vi "RES.vi"(0 "System no.":i32=1 min=1 max=4 step=1, 2 "Axes to reset":string[](array[string]), 5 "error in":errorcluster) -> (19 "error out":errorcluster)   [LabVIEW 2026]
doc: "RES (Reset Axis)\n\nDescription\nClears the \"Error\" bit (bit 0) in the status register of the axis (p. 97) and passes the axis from the \nFault state to the Ready to switch on state.\nFor further details, see \"Drive State Machine\" (p. 101). \n\nFormat\nRES <AxisID>\n\nArguments\n<AxisID>\nAn axis of the controller\nThe response to USG? CMD RES indicates in the #Related Units block for which axes the \ncommand can be used.\nPossible values: Alias of the axis (p. 94) \n\nResponse\nnone\n\nNotes\nThe status register of the axis can be queried with the STV? command (p. 66). \n\nUser command level\nUSR"
panel:
  # "RES (Reset Axis)\n\nClears the \"Error\" bit (bit 0) in the status register of the axis and passes the axis from the  Fault state to the Ready to switch on state.\nFor further details, see \"Drive State Machine\"."
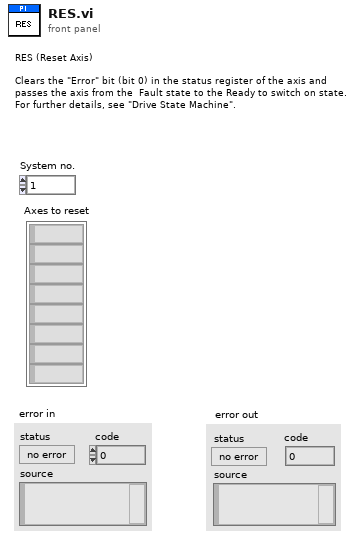
[diagram p1: front panel]
types:
  T1 = typedef "Syntax.ctl" = enum16{"GCS 1.0", "GCS 2.0", "GCS 3.0"}
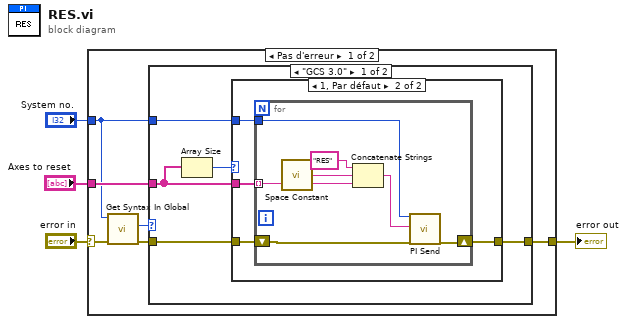
[diagram p0: block diagram]
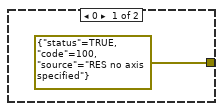
[diagram p2: hidden frame]
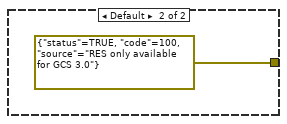
[diagram p3: hidden frame]
diagram:
  n1 = case shown="Pas d'erreur" "error in" {
    selector: "error in" -> [w8 w29]
    tunnel: [w10 w29] -> w4
    tunnel: "System no." -> [w5 _]
    tunnel: "Axes to reset" -> [w9 _]
    frame No Error {
      n2 = call "Get Syntax In Global.vi"("error in"=w8, "System no."=w5) -> ("error out"=w7:errorcluster, "Syntax"=w6:T1)  [unwired: 8 in]
      n3 = case shown="\"GCS 3.0\"" w6 {
        tunnel: [w14 errorcluster {"status"=TRUE, "code"=100, "source"="RES only available for GCS 3.0"} ("error out")] -> w10
        tunnel: w9 -> [w12 _]
        tunnel: w5 -> [w13 _]
        tunnel: w7 -> [w15 _]
        frame "GCS 3.0" {
          n4 = Array Size(array=w12) -> (size(s)=w11:i32)
          n5 = case shown="1, Par défaut" w11 {
            tunnel: w12 -> [_ w20]
            tunnel: w15 -> [_ w19]
            tunnel: [errorcluster {"status"=TRUE, "code"=100, "source"="RES no axis specified"} ("error out") w18] -> w14
            tunnel: w13 -> [_ w17]
            frame 0 {
            }
            frame 1, Default {
              n6 = for {
                tunnel: w20 -> [w24] mode=indexing
                shift-right: [w27] -> w18
                shift-left: w19 -> [w26]
                tunnel: w17 -> [w25]
                n7 = call <vilib>:"Space Constant.vi"() -> ("String"=w23:string)
                n8 = Concatenate Strings("RES", w23, w24) -> (w21:string)
                n9 = call "PI Send.vi"("System no."=w25, "String to send"=w21, "error in"=w26) -> ("error out"=w27:errorcluster)  [unwired: 3 in, 13 out]
              }
            }
          }
        }
        frame Default {
        }
      }
    }
    frame Error {
    }
  }
  "error out" <- w4
